vi "Align Visualizer.vi"(8 "Time & Dist":cluster{"Time (s)":dbl, "Distance (ft)":dbl}={"Time (s)"=0.58, "Distance (ft)"=3.664199722009253}, 11 "Points":cluster{"x":dbl, "y":dbl, "th":dbl}[](array[cluster])) -> ()   [LabVIEW 2023]
uses:
  bordeaux-pathinator/Bordeaux/Types/Segment Type.ctl
  bordeaux-pathinator/Bordeaux/Types/Trajectory Data.ctl
panel:
  in  "Time (s)":dbl(slide) scale=0.0..1.5 scale format="%#.1g"
  out "RS":bool
  in  "Sample Period (s)":dbl=0.02 min=0.001 max=1.0 format="%#_6p"
  in  "Trajectory Data":T1
  out "Picture":picture
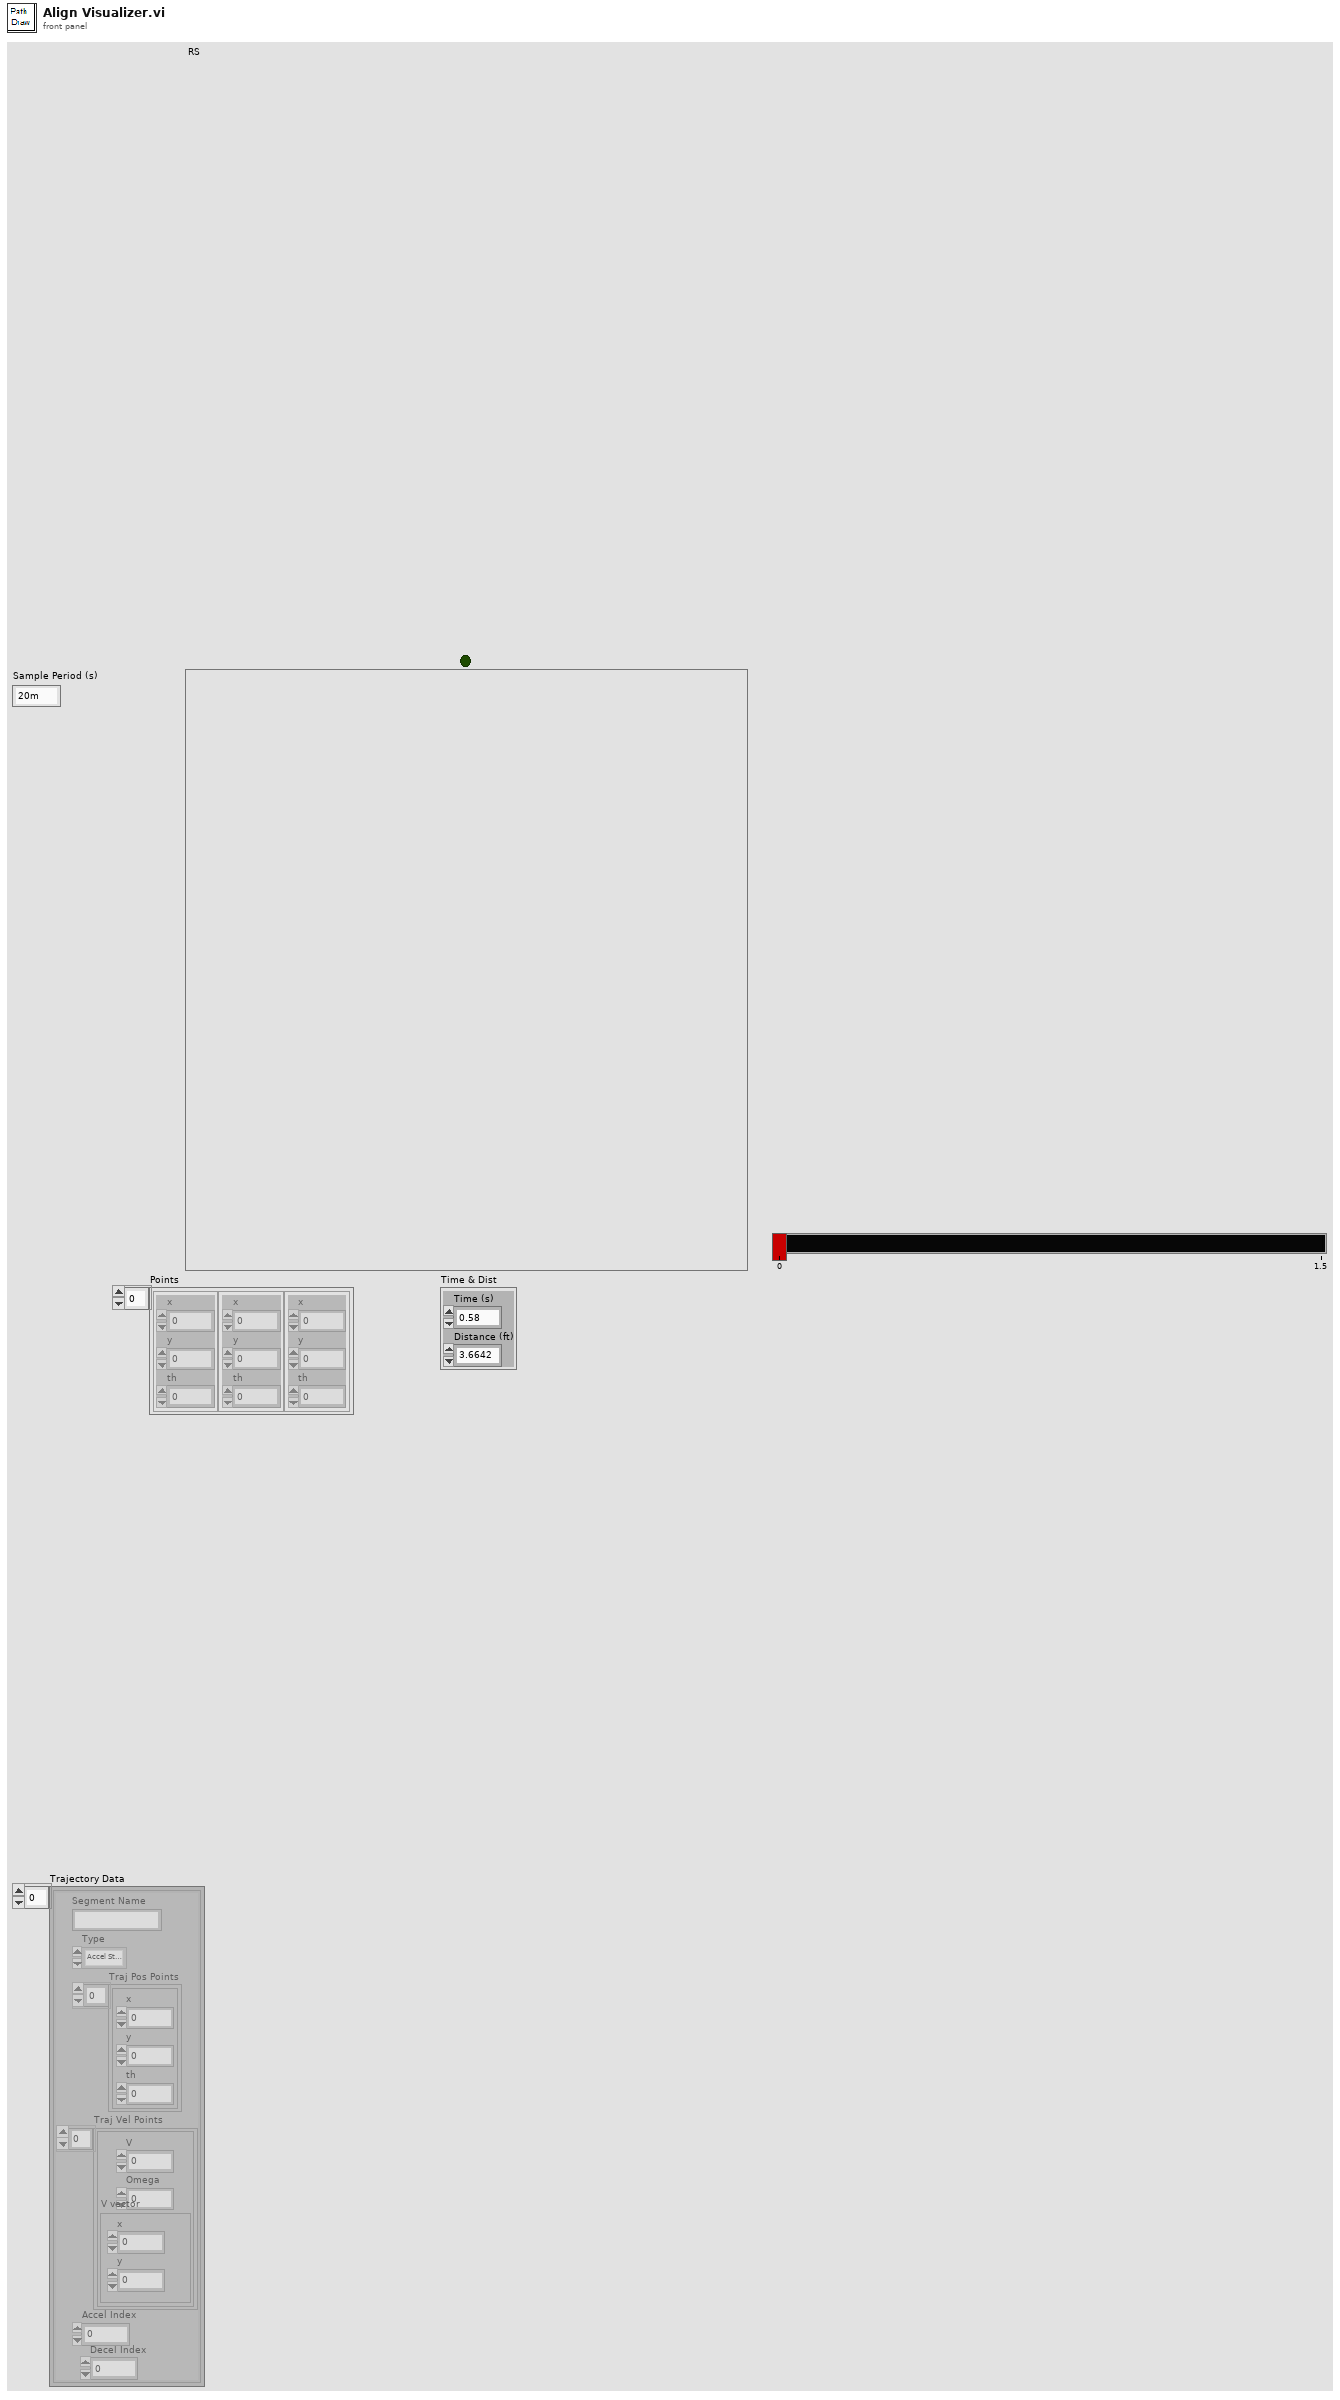
[diagram p1: front panel]
types:
  T1 = typedef "Trajectory Data.ctl" = cluster{"Segment Name":string, "Type":T2, "Traj Pos Points":cluster{"x":dbl, "y":dbl, "th":dbl}[], "Traj Vel Points":cluster{"V":dbl, "Omega":dbl, "V vector":cluster{"y":dbl, "x":dbl}}[], "Accel Index":i32, "Decel Index":i32}[]
  T2 = typedef "Segment Type.ctl" = enum16{"Accel Straight", "Const Straight", "Blend", "Circle", "Bezier"}
  T3 = cluster{"Index":i32, "Pt Test Results":enum16{"Miss", "Rect Hit", "Arrow Hit"}}
  T4 = cluster{"Horizontal":dbl, "Vertical":dbl, "th":dbl}
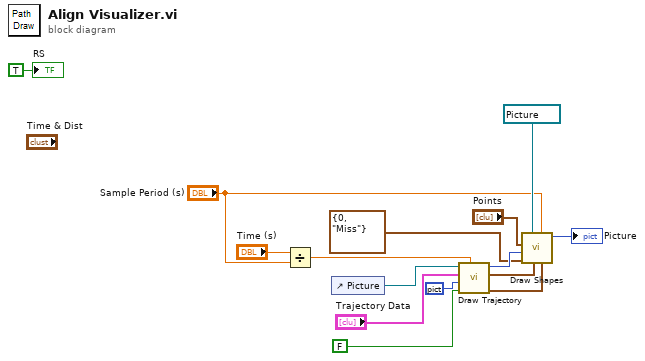
[diagram p0: block diagram]
diagram:
  n1 = Divide(x="Time (s)", y="Sample Period (s)") -> (x/y=w3:dbl)
  n2 = control-ref of="Picture"() -> (w7:refnum<vi>)
  n3 = call "Draw Trajectory.vi"("Robot Index"=w3, "Hide Path"=FALSE, "new picture in"=picture data[5B] ("new picture"), "Trajectory Data"="Trajectory Data", "Picture in"=w7) -> ("Path Points"=w12:cluster{"x":dbl, "y":dbl}[], "Output Point"=w13:T4, "new picture"=w14:picture)  [unwired: 4 in]
  n4 = call "Draw Shapes.vi"("Path Points"=w12, "Sample Period (s)"="Sample Period (s)", "Output Point"=w13, "Results"=T3 {"Index"=0, "Pt Test Results"=enum."Miss"}, "new picture in"=w14, "Points"="Points", "Picture in"=refnum<vi> refnum) -> ("new picture out"=→"Picture":picture)  [unwired: 4 in]
  "RS" <- TRUE
